vi "Telescope Debug.vi"(8 "error in (no error)":errorcluster, 10 "Debug":bool, 11 "LDT Telescope in":refnum<class "LDT Telescope.lvclass">) -> (0 "error out":errorcluster, 3 "LDT Telescope out":refnum<class "LDT Telescope.lvclass">)   [LabVIEW 2022 SP3, in "LDT Telescope.lvclass"]
uses:
  LDT Telescope.lvclass
  LDT Telescope.lvclass/LDT Telescope.ctl
  Telescope.lvclass
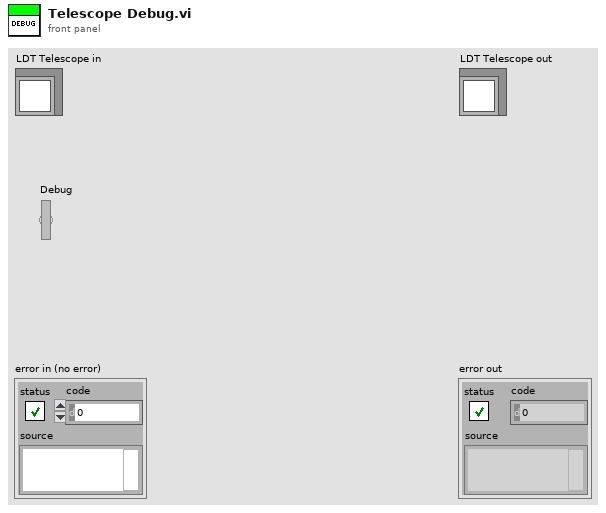
[diagram p1: front panel]
types:
  T1 = enum32{"Invalid", "Standard", "Closed", "Hidden", "Minimized", "Maximized"}
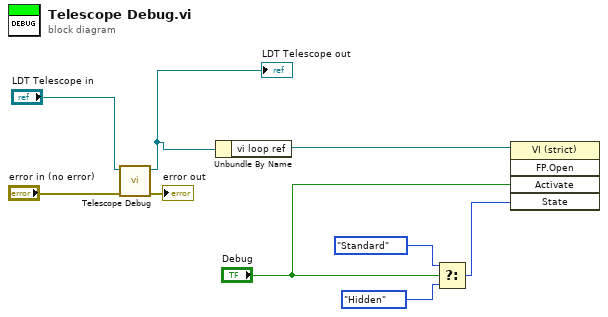
[diagram p0: block diagram]
diagram:
  n1 = call-parent "Telescope Debug.vi"("error in (no error)"="error in (no error)", "Telescope in"="LDT Telescope in") -> ("error out"=→"error out":errorcluster, "Telescope out"=w6:refnum<class "LDT Telescope.lvclass">)  [unwired: 8 in]
  "LDT Telescope out" <- w6
  n2 = Unbundle By Name(w6) -> ("vi loop ref"=w3:refnum<vi>)
  n3 = Select(t=T1."Standard" ("Front Panel Window:State"), s="Debug", f=T1."Hidden" ("Front Panel Window:State")) -> (s? t:f=w2:T1)
  n4 = invoke class="VI (strict)" method="FP.Open"(reference=w3, "Activate"="Debug", "State"=w2) -> ()  [unwired: 2 in, 5 out]
